vi "DAQmx-AI.FindSelectedDevice.vi"(8 "error in (no error)":errorcluster, 11 "Device Name":tag="SMO-Sim") -> (0 "error out":errorcluster, 1 "Simulated":bool, 2 "Device found":bool, 3 "ActiveDev":tag="SMO-Sim")   [LabVIEW 2016, in "DAQmx-AI.lvclass"]
uses:
  DAQmx-AI.lvclass
  <resource>/objmgr/daqmx.rc
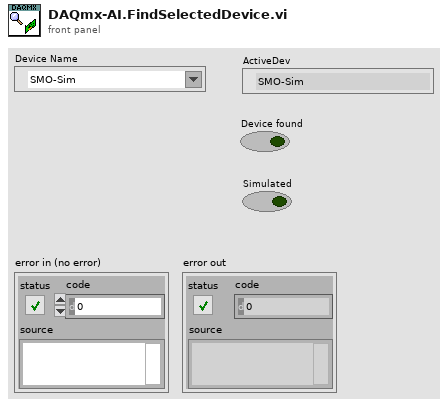
[diagram p1: front panel]
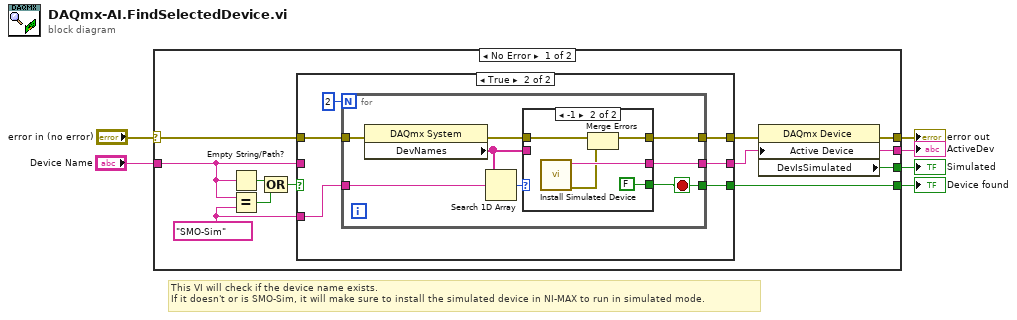
[diagram p0: block diagram]
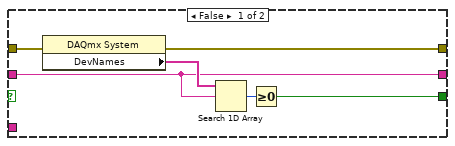
[diagram p2: hidden frame]
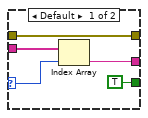
[diagram p3: hidden frame]
diagram:
  # "This VI will check if the device name exists.\nIf it doesn't or is SMO-Sim, it will make sure to install the simulated device in NI-MAX to run in simulated mode."
  n1 = case shown="No Error" "error in (no error)" {
    selector: "error in (no error)" -> [w12 w49]
    tunnel: [w17 _] -> w6
    tunnel: [w10 w48] -> w5
    tunnel: [w16 _] -> w4
    tunnel: "Device Name" -> [w9 w48]
    tunnel: [w13 w49] -> w2
    frame No Error {
      w7 = tag "SMO-Sim" ("ActiveDev")
      n2 = Empty String/Path?(string/path=w9) -> (empty?=w15:bool)
      n3 = Equal?(x=w9, y=w7) -> (x = y?=w8:bool)
      n4 = Compound Arithmetic op=OR(w15, w8) -> (w14:bool)
      n5 = case shown="True" w14 {
        tunnel: w9 -> [w22 _]
        tunnel: [w21 w29] -> w17
        tunnel: [w22 w27] -> w10
        tunnel: w12 -> [w18 w25]
        tunnel: [w19 w24] -> w11
        tunnel: w7 -> [_ w26]
        frame False {
          n6 = property class="DAQmx System"(error in=w18) -> (error out=w19:errorcluster, "DevNames"=w23:tag[])  [unwired: 1 in, 1 out]
          n7 = Search 1D Array(1D array=w23, element=w22) -> (index of element=w20:i32)  [unwired: 1 in]
          n8 = Greater Or Equal To 0?(x=w20) -> (x >= 0?=w21:bool)
        }
        frame True {
          n9 = for {
            N: 2 -> [_]
            tunnel: [w36] -> w27
            tunnel: [w35] -> w29
            tunnel: w26 -> [w32]
            tunnel: w25 -> [w31]
            tunnel: [w30] -> w24
            stop <- w35 stop-if-true
            n10 = property class="DAQmx System"(error in=w31) -> (error out=w33:errorcluster, "DevNames"=w34:tag[])  [unwired: 1 in, 1 out]
            n11 = Search 1D Array(1D array=w34, element=w32) -> (index of element=w37:i32)  [unwired: 1 in]
            n12 = case shown="-1" w37 {
              selector: w37 -> [w41 _]
              tunnel: w34 -> [w42 _]
              tunnel: [w40 w46] -> w36
              tunnel: [TRUE FALSE] -> w35
              tunnel: w33 -> [w38 w44]
              tunnel: [w38 w43] -> w30
              frame Default {
                n13 = Index Array(array=w42, index=w41) -> (element=w40:tag)
              }
              frame -1 {
                n14 = call "Install Simulated Device.vi"() -> ("error out"=w45:errorcluster, "Device Name"=w46:tag)  [unwired: 10 in]
                n15 = Merge Errors(w44, w45) -> (w43:errorcluster)
              }
            }
          }
        }
      }
      n16 = property class="DAQmx Device"(error in=w11, "Active Device"=w10) -> (error out=w13:errorcluster, "DevIsSimulated"=w16:bool)  [unwired: 1 in, 1 out]
    }
    frame Error {
    }
  }
  "ActiveDev" <- w5
  "Device found" <- w6
  "error out" <- w2
  "Simulated" <- w4
